vi "Event Handle Loop_Call Pop-out Panel.vi"(8 "error in (no error)":errorcluster, 11 "QTab Class in":refnum<class "QTab Class.lvclass">) -> (0 "error out":errorcluster, 3 "QTab Class out":refnum<class "QTab Class.lvclass">)   [LabVIEW 2020, in "QTab.lvlib" / "QTab Class.lvclass"]
uses:
  QTab Class.lvclass
  Event Handle Loop_Pop-out Panel.vi
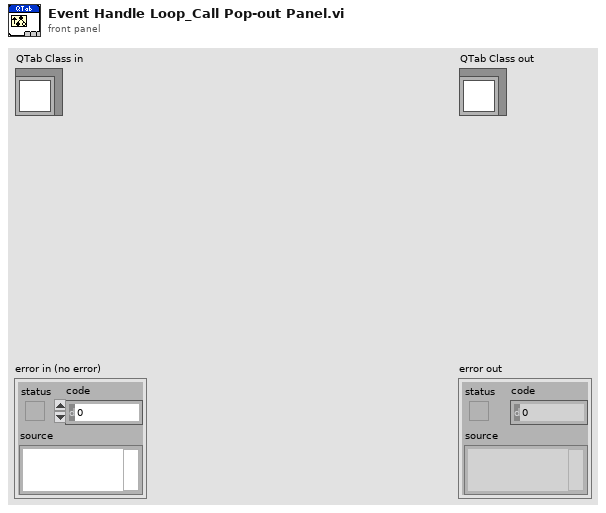
[diagram p1: front panel]
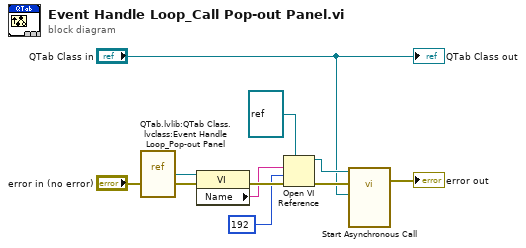
[diagram p0: block diagram]
diagram:
  n1 = vi-ref "QTab.lvlib:QTab Class.lvclass:Event Handle Loop_Pop-out Panel.vi"() -> (w10:refnum<vi>)
  n2 = property class="VI"(reference=w10, error in="error in (no error)") -> (error out=w9:errorcluster, "Name"=w8:string)  [unwired: 1 out]
  n3 = Open VI Reference(type specifier VI Refnum (for type only)=refnum<vi> refnum, vi path=w8, options=192 ("timeout ms (60000)"), error in (no error)=w9) -> (vi reference=w4:refnum<vi>, error out=w6:errorcluster)  [unwired: 2 in]
  n4 = call-by-ref "Start Asynchronous Call"(reference=w4, error in=w6, "QTab Class in"="QTab Class in") -> (error out=→"error out":errorcluster)  [unwired: 10 in, 2 out]
  "QTab Class out" <- "QTab Class in"
